vi "SP Create Limit Spec.vi"(4 "Limit":T1[](array[typedef])) -> (1 "Limit Traces":cluster{"X":dbl[], "Y":dbl[]}[](array[cluster]))   [LabVIEW 2011]
uses:
  TypeDefs/SP Limit Point.ctl
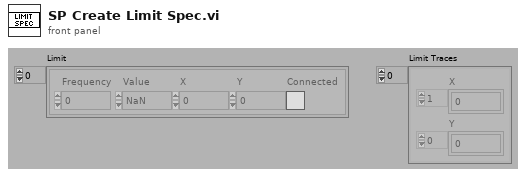
[diagram p1: front panel]
types:
  T1 = typedef "SP Limit Point.ctl" = cluster{"Frequency":dbl, "Value":dbl, "X":dbl, "Y":dbl, "Connected":bool}
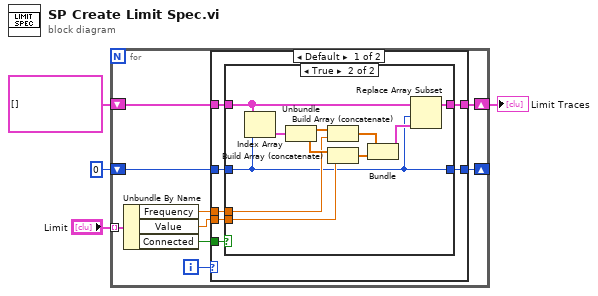
[diagram p0: block diagram]
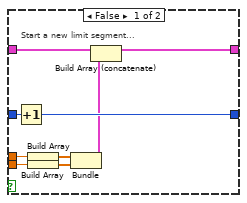
[diagram p2: hidden frame]
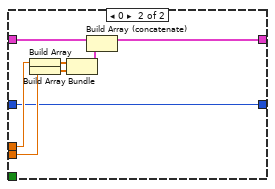
[diagram p3: hidden frame]
diagram:
  n1 = for {
    shift-right: [w9] -> w3
    shift-left: cluster{"X":dbl[], "Y":dbl[]}[] [] ("Limit Specification") -> [w12]
    tunnel: "Limit" -> [w13] mode=indexing
    shift-right: [w7] -> _
    shift-left: 0 -> [w8]
    i -> [w5]
    n2 = Unbundle By Name(w13) -> ("Frequency"=w11:dbl, "Value"=w6:dbl, "Connected"=w10:bool)
    n3 = case shown="Default" w5 {
      tunnel: w12 -> [w16 w46]
      tunnel: w11 -> [w19 w48]
      tunnel: w6 -> [w18 w47]
      tunnel: w10 -> [w20 _]
      tunnel: [w14 w42] -> w9
      tunnel: w8 -> [w17 w41]
      tunnel: [w15 w41] -> w7
      frame Default {
        n4 = case shown="True" w20 {
          tunnel: w19 -> [w25 w37]
          tunnel: w18 -> [w21 w36]
          tunnel: w17 -> [w27 w31]
          tunnel: w16 -> [w29 w33]
          tunnel: [w26 w31] -> w15
          tunnel: [w28 w30] -> w14
          frame False {
            # "Start a new limit segment..."
            n5 = Increment(x=w27) -> (x+1=w26:i32)
            n6 = Build Array(w25) -> (w24:dbl[])
            n7 = Build Array(w21) -> (w23:dbl[])
            n8 = Bundle(w24, w23) -> (w22:cluster{dbl[], dbl[]})  [unwired: 1 out]
            n9 = Build Array (concatenate)(w29, w22) -> (w28:cluster{"X":dbl[], "Y":dbl[]}[])
          }
          frame True {
            n10 = Index Array(array=w33, index=w31) -> (element=w40:cluster{"X":dbl[], "Y":dbl[]})
            n11 = Unbundle(w40) -> ("X"=w39:dbl[], "Y"=w38:dbl[])
            n12 = Build Array (concatenate)(w39, w37) -> (w35:dbl[])
            n13 = Build Array (concatenate)(w38, w36) -> (w34:dbl[])
            n14 = Bundle(w35, w34) -> (w32:cluster{dbl[], dbl[]})  [unwired: 1 out]
            n15 = Replace Array Subset(array=w33, new element=w32, index=w31) -> (w30:cluster{"X":dbl[], "Y":dbl[]}[])
          }
        }
      }
      frame 0 {
        n16 = Build Array(w48) -> (w45:dbl[])
        n17 = Build Array(w47) -> (w44:dbl[])
        n18 = Bundle(w45, w44) -> (w43:cluster{dbl[], dbl[]})  [unwired: 1 out]
        n19 = Build Array (concatenate)(w46, w43) -> (w42:cluster{"X":dbl[], "Y":dbl[]}[])
      }
    }
  }
  "Limit Traces" <- w3
